vi "DriveModuleControl_TravTunePID.vi"(8 "error in":errorcluster, 9 "Actual State":T1={"Speed"=0.0, "Angle"={"VALUE"=0.0, "COS"=1.0, "SIN"=0.0}} {"Angle"."SIN" format="%13.4f"; "Angle"."COS" format="%13.4f"; "Angle"."VALUE" format="%13.4f"}, 10 "Desired State":T1={"Speed"=0.0, "Angle"={"VALUE"=0.0, "COS"=1.0, "SIN"=0.0}} {"Angle"."SIN" format="%13.4f"; "Angle"."COS" format="%13.4f"; "Angle"."VALUE" format="%13.4f"}, 11 "ModualNamePrefix":i32) -> (0 "error out":errorcluster)   [LabVIEW 2023]
uses:
  <vilib>/Rock Robotics/WPI/ThirdParty/JAS_Junk/TrajLib/TypeDef/SWERVE_DRIVE_MODULE_STATE.ctl
  <vilib>/Rock Robotics/WPI/ThirdParty/JAS_Junk/TrajLib/TypeDef/ROTATION2D.ctl
  <vilib>/Rock Robotics/WPI/ThirdParty/JAS_Junk/TrajLib/Rotation2d_Minus.vi
  <vilib>/Rock Robotics/WPI/ThirdParty/JAS_Junk/TrajLib/Rotation2d_GetRadians.vi
  <vilib>/Rock Robotics/WPI/ThirdParty/JAS_Junk/TrajLib/SwerveModuleState_New.vi
  <vilib>/Rock Robotics/WPI/ThirdParty/JAS_Junk/TrajLib/Rotation2d_RotateBy.vi
  <vilib>/Rock Robotics/WPI/ThirdParty/JAS_Junk/TrajLib/Rotation2d_CreateAngle.vi
  <vilib>/Rock Robotics/WPI/ThirdParty/JAS_Junk/TrajLib/Timer_New.vi
  <vilib>/Rock Robotics/WPI/ThirdParty/JAS_Junk/TrajLib/SimpleMotorFF_Calculate.vi
  <vilib>/Rock Robotics/WPI/ThirdParty/JAS_Junk/TrajLib/PIDController_AtSetpoint.vi
  <vilib>/Rock Robotics/WPI/ThirdParty/JAS_Junk/TrajLib/PIDController_SetPIDF.vi
  <vilib>/Rock Robotics/WPI/ThirdParty/JAS_Junk/TrajLib/PIDController_SetDerivativeFilter.vi
  <vilib>/Rock Robotics/WPI/ThirdParty/JAS_Junk/TrajLib/PIDController_SetIntegratorRange.vi
  <vilib>/Rock Robotics/WPI/ThirdParty/JAS_Junk/TrajLib/PIDController_SetTolerancePandV.vi
  <vilib>/Rock Robotics/WPI/ThirdParty/JAS_Junk/TrajLib/PIDController_DisableContinousInput.vi
  <vilib>/Rock Robotics/WPI/ThirdParty/JAS_Junk/TrajLib/PIDController_EnableContinousInput.vi
  <vilib>/Rock Robotics/WPI/ThirdParty/JAS_Junk/TrajLib/PIDController_Reset.vi
  <vilib>/Rock Robotics/WPI/ThirdParty/JAS_Junk/TrajLib/PIDController_New.vi
  <vilib>/Rock Robotics/WPI/ThirdParty/JAS_Junk/TrajLib/PIDController_SetOutputLimits.vi
  <vilib>/Rock Robotics/WPI/ThirdParty/JAS_Junk/TrajLib/VI/PIDController_SetIntegratorZone.vi
  <vilib>/Rock Robotics/WPI/ThirdParty/JAS_Junk/TrajLib/Rotation2d_UnaryMinus.vi
  <vilib>/Rock Robotics/WPI/ThirdParty/JAS_Junk/TrajLib/Rotation2d_CreateXY.vi
  <vilib>/Rock Robotics/WPI/ThirdParty/JAS_Junk/TrajLib/PIDController_NewPeriod.vi
  <vilib>/Rock Robotics/WPI/ThirdParty/JAS_Junk/TrajLib/Util_CalcDist.vi
  <vilib>/Rock Robotics/SystemInterfaces/NetworkCommunication/NetComm_UsageReport_report.vi
  <vilib>/Rock Robotics/WPI/ThirdParty/Phoenix6/Phoenix6_Device_RefNumRegistryGet.vi
  <vilib>/Rock Robotics/WPI/MotorControl/WPI_MotorControlRefNum Registry Get.vi
  <vilib>/Rock Robotics/Network Tables/NT Write Number.vi
  <vilib>/Utility/semaphor.llb/Obtain Semaphore Reference.vi
  <vilib>/Rock Robotics/WPI/ThirdParty/JAS_Junk/TrajLib/Timer_Reset.vi
  <vilib>/Rock Robotics/WPI/ThirdParty/JAS_Junk/TrajLib/Timer_Start.vi
  <vilib>/Rock Robotics/WPI/ThirdParty/JAS_Junk/TrajLib/Timer_Stop.vi
  <vilib>/Rock Robotics/WPI/ThirdParty/JAS_Junk/TrajLib/Timer_HasPeriodPassedOnce.vi
  DriveGlobal.vi
  <vilib>/Rock Robotics/WPI/ThirdParty/JAS_Junk/TrajLib/Globals/Util_LibraryGlobals.vi
  <vilib>/Rock Robotics/WPI/ThirdParty/JAS_Junk/TrajLib/PIDController_AdvCalculate_FF_Sp_Pv.vi
  DriveTuningGlobals.vi
  <vilib>/Rock Robotics/WPI/ThirdParty/JAS_Junk/TrajLib/Trajectory_Library.lvlib
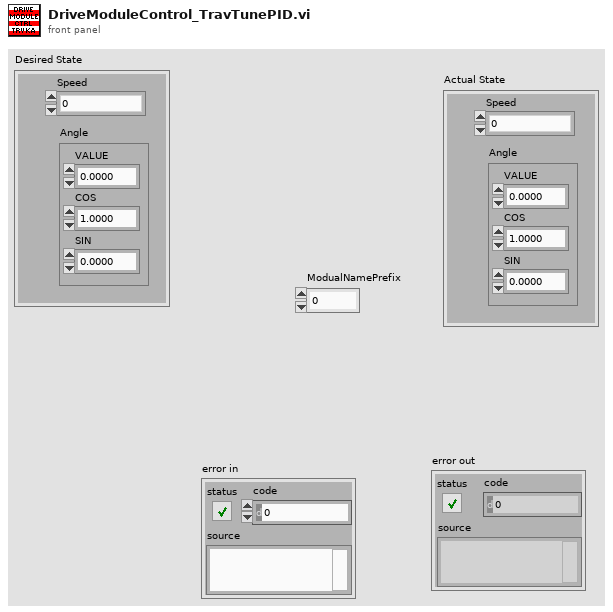
[diagram p1: front panel]
types:
  T1 = typedef "Trajectory_Library.lvlib/SWERVE_DRIVE_MODULE_STATE.ctl" = cluster{"Speed":dbl, "Angle":T2}
  T2 = typedef "Trajectory_Library.lvlib/ROTATION2D.ctl" = cluster{"VALUE":dbl, "COS":dbl, "SIN":dbl}
  T3 = enum16{"Ziegler Nicols - Fast", "Ziegler Nicols - Normal", "Ziegler Nicols - Slow", "CHR regulator - 0% overshoot", "CHR regulator - 20% overshoot", "CHR servo - 0 % overshoot", "CHR servo - 20% overshoot"}
  T4 = typedef "WPI_MotorControlDeviceRef.ctl" = cluster{"DeviceStatus":errorcluster, "Type":T5, "PWM":cluster{"PWM Channel":T6, "DeadBand":T7}, "CAN":cluster{"Device Number":u8, "SetOutput VI Ref":variant, "GetOutput VI Ref":variant, "Enable VI Ref":variant, "Disable VI Ref":variant, "Data":variant}, "Invert":bool, "DIO PWM":cluster{"PWM \"Enable\" Channel":T6, "DIOChannel":T8, "PWM Rate":dbl}}
  T5 = typedef "WPI_MotorControlType.ctl" = enum16{"PWM", "CAN", "DIO PWM"}
  T6 = typedef "FPGA_DIOPWMChannel.ctl" = enum8{"PWM 0", "PWM 1", "PWM 2", "PWM 3", "PWM 4", "PWM 5", "PWM 6", "PWM 7", "PWM 8", "PWM 9", "PWM MXP 0", "PWM MXP 1", "PWM MXP 2", "PWM MXP 3", "PWM MXP 4", "PWM MXP 5", "PWM MXP 6", "PWM MXP 7", "PWM MXP 8", "PWM MXP 9", "Invalid"}
  T7 = typedef "WPI_PWMDeadband.ctl" = cluster{"Name":string, "maxPositivePwm":i32, "minPositivePwm":i32, "centerPwm":i32, "maxNegativePwm":i32, "minNegativePwm":i32, "angularRange":u16}
  T8 = typedef "FPGA_DIOChannel.ctl" = enum8{"DIO 0", "DIO 1", "DIO 2", "DIO 3", "DIO 4", "DIO 5", "DIO 6", "DIO 7", "DIO 8", "DIO 9", "DIO MXP 0", "DIO MXP 1", "DIO MXP 2", "DIO MXP 3", "DIO MXP 4", "DIO MXP 5", "DIO MXP 6", "DIO MXP 7", "DIO MXP 8", "DIO MXP 9", "DIO MXP 10", "DIO MXP 11", "DIO MXP 12", "DIO MXP 13", "DIO MXP 14", "DIO MXP 15", "SPI Port CS1", "SPI Port CS2", "SPI Port CS3", "SPI Port MISO", "SPI Port MOSI", "Invalid"}
  T9 = typedef "Trajectory_Library.lvlib/SIMPLE_MOTOR_FF.ctl" = cluster{"Ks":dbl, "Kv":dbl, "Ka":dbl, "KnInv":dbl}
  T10 = typedef "Trajectory_Library.lvlib/PID_ADV_LIMITS.ctl" = cluster{"MaxInput":dbl, "MinInput":dbl, "Continuous":bool, "MaxOutput":dbl, "MinOutput":dbl}
  T11 = typedef "Trajectory_Library.lvlib/PID_ADV_TUNING.ctl" = cluster{"Kf":dbl, "Kp":dbl, "Ki":dbl, "Kd":dbl, "MaximumIntegral":dbl, "MinimumIntegral":dbl, "Filter Derivative":bool, "IntegralZone":dbl}
  T12 = cluster{"Controller Constant Type":enum16{"Ziegler Nicols - Fast", "Ziegler Nicols - Normal", "Ziegler Nicols - Slow", "CHR regulator - 0% overshoot", "CHR regulator - 20% overshoot", "CHR servo - 0 % overshoot", "CHR servo - 20% overshoot"}, "Type of Controller":enum16{"P", "PI", "PID"}, "CO Offset":dbl, "Kn":dbl, "Tuning Tolerance":dbl, "Plant Tolerance":dbl, "Newest Avg Time ":i32, "Long Ave Time":i32}
  T13 = cluster{"Plant Gain (K)":dbl, "Time Constant (T)":dbl, "Dead Time (L)":dbl, "stimulus operating point":dbl, "response operating point":dbl}
  T14 = cluster{"proportional gain (Kp)":dbl, "integral time (Ki / Sec)":dbl, "derivative time (Kd /Sec)":dbl}
  T15 = cluster{"Const Done":bool, "Plant Done":bool, "PV Std Dev":dbl, "CO Std Dev":dbl}
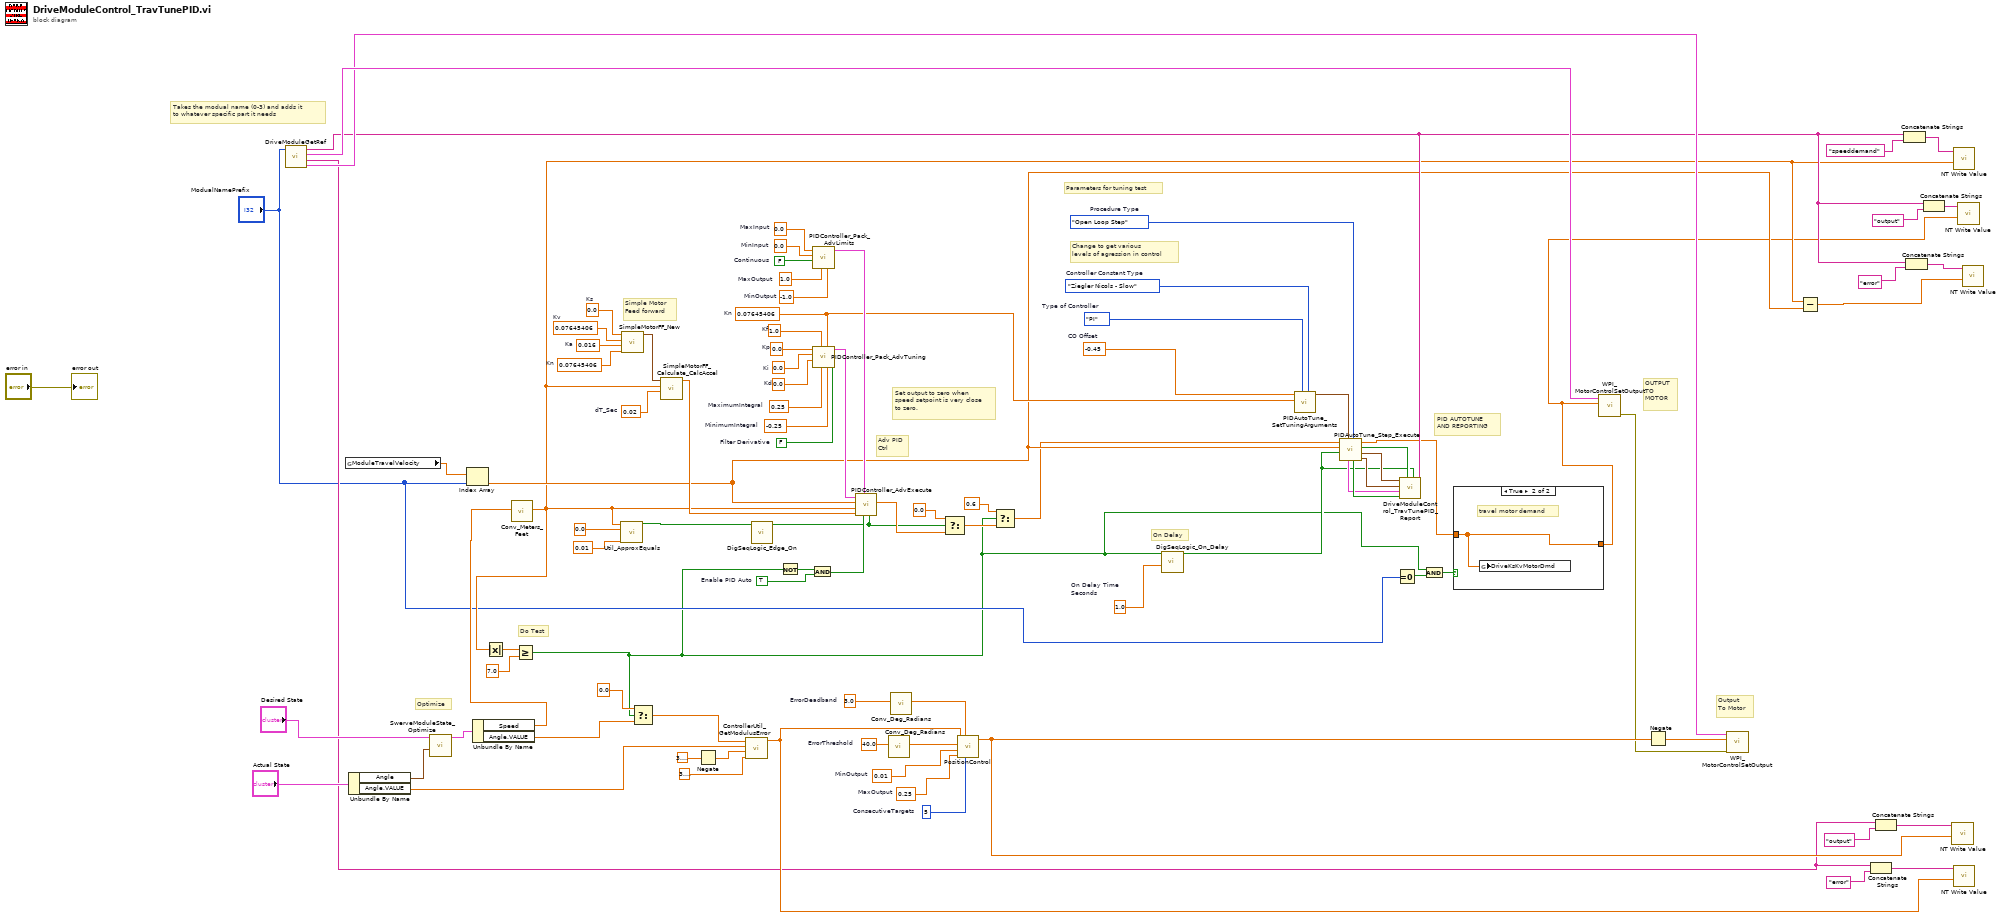
[diagram p0: block diagram]
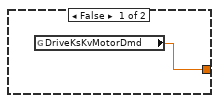
[diagram p2: hidden frame]
diagram:
  w10 = 1.0  # On Delay Time Seconds
  w23 = enum16{"Open Loop Step", "Closed Loop Step"}."Open Loop Step"  # Procedure Type
  w24 = T3."Ziegler Nicols - Slow"  # Controller Constant Type
  w25 = enum16{"P", "PI", "PID"}."PI"  # Type of Controller
  w26 = -0.45  # CO Offset
  w36 = TRUE  # Enable PID Auto
  w22 = 0.07645406  # Kn
  w60 = 0.0  # Kp
  w59 = 0.0  # Ki
  w58 = 0.0  # Kd
  w57 = 1.0  # Kf
  w56 = 0.25  # MaximumIntegral
  w55 = -0.25  # MinimumIntegral
  w54 = FALSE  # Filter Derivative
  w52 = 0.0  # MinInput
  w51 = FALSE  # Continuous
  w50 = 1.0  # MaxOutput
  w53 = -1.0  # MinOutput
  w49 = 0.0  # MaxInput
  w69 = 0.07645406  # Kn
  w68 = 0.02  # dT_Sec
  w66 = 0.0  # Ks
  w65 = 0.07645406  # Kv
  w64 = 0.016  # Ka
  w79 = 5  # ConsecutiveTargets
  w76 = 0.25  # MaxOutput
  w80 = 0.01  # MinOutput
  w73 = 40.0  # ErrorThreshold
  w75 = 3.0  # ErrorDeadband
  # "On Delay"
  # "Output\nTo Motor"
  # "OUTPUT\nTO \nMOTOR"
  # "PID AUTOTUNE\nAND REPORTING"
  # "Change to get various\nlevels of agression in control"
  # "Parameters for tuning test"
  # "Do Test"
  # "Optimize"
  # "Set output to zero when\nspeed setpoint is very close\nto zero."
  # "Adv PID\nCtrl"
  # "Simple Motor\nFeed forward"
  # "Takes the modual name (0-3) and adds it \nto whatever specific part it needs"
  n1 = call "DriveModuleGetRef.vi"("ModualNamePrefix"="ModualNamePrefix") -> ("SpinMot"=w61:T4, "SpinStr"=w41:string, "TravMot"=w62:T4, "TravStr"=w18:string)  [unwired: 5 in, 2 out]
  n2 = global read "DriveGlobal.vi" "ModuleTravelVelocity"() -> (w45:dbl[])
  n3 = Unbundle By Name("Actual State") -> ("Angle"=w86:T2, "Angle.VALUE"=w83:dbl)
  n4 = call <vilib>:"SwerveModuleState_Optimize.vi"("CurrentAngle"=w86, "Desired State"="Desired State") -> ("out SWERVE_DRIVE_MODULE_STATE"=w84:T1)  [unwired: 9 in]
  n5 = Index Array(array=w45, index="ModualNamePrefix") -> (element=w15:dbl)
  n6 = Unbundle By Name(w84) -> ("Speed"=w33:dbl, "Angle.VALUE"=w30:dbl)
  n7 = call <vilib>:"Conv_Meters_Feet.vi"("Meters"=w33) -> ("Feet"=w14:dbl)  [unwired: 10 in]
  n8 = Absolute Value(x=w14) -> (abs(x)=w32:dbl)
  n9 = Greater Or Equal?(x=w32, y=7.0) -> (x >= y?=w3:bool)
  n10 = call <vilib>:"Util_ApproxEquals.vi"("Tolerance"=0.01, "Value 2"=0.0, "Value 1"=w14) -> ("ApproxEquals"=w2:bool)  [unwired: 8 in]
  n11 = call <vilib>:"SimpleMotorFF_New.vi"("Kn"=w69, "Ka"=w64, "Kv"=w65, "Ks"=w66) -> ("SIMPLE_MOTOR_FF"=w67:T9)  [unwired: 7 in]
  n12 = Select(t=0.0, s=w3, f=w30) -> (s? t:f=w28:dbl)
  n13 = call <vilib>:"SimpleMotorFF_Calculate_CalcAccel.vi"("dT_Sec"=w68, "VelSp"=w14, "SIMPLE_MOTOR_FF"=w67) -> ("FeedForward"=w46:dbl)  [unwired: 8 in]
  n14 = Negate(x=3.141592653589793) -> (-x=w85:dbl)
  n15 = call <vilib>:"ControllerUtil_GetModulusError.vi"("Maximum_Input"=3.141592653589793, "Minimum_Input"=w85, "Measurerment(PV)"=w83, "Reference(SP)"=w28) -> ("Error"=w77:dbl)  [unwired: 7 in]
  n16 = call <vilib>:"DigSeqLogic_Edge_On.vi"("Input"=w2) -> ("On Edge"=w1:bool)  [unwired: 10 in]
  n17 = Not(x=w3) -> (.not. x?=w37:bool)
  n18 = And(x=w37, y=w36) -> (x .and. y?=w38:bool)
  n19 = call <vilib>:"PIDController_Pack_AdvLimits.vi"("MinOutput"=w53, "MaxOutput"=w50, "Continuous"=w51, "MinInput"=w52, "MaxInput"=w49) -> ("Adv PID Limits"=w47:T10)  [unwired: 6 in]
  n20 = call <vilib>:"PIDController_Pack_AdvTuning.vi"("Filter Derivative"=w54, "MinimumIntegral"=w55, "Kn"=w22, "MaximumIntegral"=w56, "Kf"=w57, "Kd"=w58, "Ki"=w59, "Kp"=w60) -> ("Adv PID Tuning"=w48:T11)  [unwired: 3 in]
  n21 = call <vilib>:"PIDController_AdvExecute.vi"("Reset"=w1, "Auto"=w38, "Adv PID Limits"=w47, "FF-FeedForward"=w46, "SP-SetPoint"=w14, "PV-Measurement"=w15, "Adv PID Tuning"=w48) -> ("CO-ControlOutput"=w35:dbl)  [unwired: 2 in, 2 out]
  n22 = call <vilib>:"Conv_Deg_Radians.vi"("Degress"=w73) -> ("Radians"=w72:dbl)  [unwired: 10 in]
  n23 = call <vilib>:"Conv_Deg_Radians.vi"("Degress"=w75) -> ("Radians"=w74:dbl)  [unwired: 10 in]
  n24 = Select(t=0.0, s=w1, f=w35) -> (s? t:f=w13:dbl)
  n25 = call "PositionControl.vi"("ConsecutiveTargets"=w79, "ErrorDeadband"=w74, "MaxOutput"=w76, "MinOutput"=w80, "ErrorThreshold"=w72, "Error"=w77) -> ("OutputValue"=w71:dbl)  [unwired: 3 in, 2 out]
  n26 = Select(t=0.6, s=w3, f=w13) -> (s? t:f=w12:dbl)
  n27 = call <vilib>:"DigSeqLogic_On_Delay.vi"("Delay"=w10, "Input"=w3) -> ("Output"=w9:bool)  [unwired: 8 in, 1 out]
  n28 = call <vilib>:"PIDAutoTune_SetTuningArguments.vi"("Controller Constant Type"=w24, "Type of Controller"=w25, "Kn"=w22, "CO Offset"=w26) -> ("Configuration Parameters"=w27:T12)  [unwired: 7 in]
  n29 = call <vilib>:"PIDAutoTune_Step_Execute.vi"("Procedure Type"=w23, "Configuration Parameters"=w27, "Tune"=w9, "Measurement  (PV)"=w15, "Control Output (Co)"=w12) -> ("Plant and Test Data"=w20:T13, "New Tuning Parameters"=w21:T14, "Tuning Done"=w19:bool, "Adj CO"=w8:dbl, "Error Occured"=w17:bool, "Diagnostic Info"=w16:T15)  [unwired: 1 in]
  n30 = Equal To 0?(x="ModualNamePrefix") -> (x = 0?=w4:bool)
  n31 = call "DriveModuleControl_TravTunePID_Report.vi"("Network Table Prefix"=w18, "TestInProgress"=w9, "Tuning Done"=w19, "Error Occured"=w17, "Diagnostic Info"=w16, "Plant and Test Data"=w20, "New Tuning Parameters"=w21) -> ()  [unwired: 5 in]
  n32 = And(x=w3, y=w4) -> (x .and. y?=w5:bool)
  n33 = case shown="True" w5 {
    tunnel: [w97 w98] -> w7
    tunnel: w8 -> [_ w98]
    frame False {
      n34 = global read "DriveTuningGlobals.vi" "DriveKsKvMotorDmd"() -> (w97:dbl)
    }
    frame True {
      # "travel motor demand"
      n35 = global write "DriveTuningGlobals.vi" "DriveKsKvMotorDmd"(w98) -> ()
    }
  }
  n36 = call <vilib>:"WPI_MotorControlSetOutput.vi"("Output"=w7, "MotorControlDevRef"=w62) -> ("error out"=w63:errorcluster)  [unwired: 7 in, 2 out]
  n37 = Negate(x=w71) -> (-x=w70:dbl)
  n38 = call <vilib>:"WPI_MotorControlSetOutput.vi"("error in (no error)"=w63, "Output"=w70, "MotorControlDevRef"=w61) -> ()  [unwired: 6 in, 3 out]
  n39 = Subtract(x=w14, y=w15) -> (x-y=w42:dbl)
  n40 = Concatenate Strings(w41, "error" ("refnum name")) -> (w90:string)
  n41 = Concatenate Strings(w41, "output" ("refnum name")) -> (w78:string)
  n42 = Concatenate Strings(w18, "speeddemand" ("refnum name")) -> (w94:string)
  n43 = Concatenate Strings(w18, "error" ("refnum name")) -> (w43:string)
  n44 = Concatenate Strings(w18, "output" ("refnum name")) -> (w92:string)
  n45 = call-poly <vilib>:"NT Write Value.vi"("value"=w71, "name"=w78) -> ()  [unwired: 9 in, 1 out]
  n46 = call-poly <vilib>:"NT Write Value.vi"("value"=w14, "name"=w94) -> ()  [unwired: 9 in, 1 out]
  n47 = call-poly <vilib>:"NT Write Value.vi"("value"=w77, "name"=w90) -> ()  [unwired: 9 in, 1 out]
  n48 = call-poly <vilib>:"NT Write Value.vi"("value"=w7, "name"=w92) -> ()  [unwired: 9 in, 1 out]
  n49 = call-poly <vilib>:"NT Write Value.vi"("value"=w42, "name"=w43) -> ()  [unwired: 9 in, 1 out]
  "error out" <- "error in"
